vi "PID engine.vi"(0 "Temp In (deg C)":dbl format="%.2f", 7 "Control Parameters":T1={"Setpoint"=50.0, "Control bandwidth"=4.0, "Settle bandwidth"=1.0, "Integral time"=30.0, "Int\non"=TRUE, "Derivative time"=0.5, "Der\non"=FALSE, "Settle time"=200.0} {"Settle time" format="%.2f"; "Derivative time" format="%.2f"; "Integral time" format="%.2f"; "Settle bandwidth" format="%.2f"; "Control bandwidth" format="%.2f"; "Setpoint" format="%.2f"}, 11 "error in":errorcluster, 12 "Normalized Power In (0-1)":dbl format="%.2f", 13 "index (0=init)":i32, 14 "Manual Override":bool) -> (2 "settled":bool, 3 "time in settle band":dbl format="%.2f", 4 "Normalized Power Out (0-1)":dbl format="%.2f", 15 "error out":errorcluster)   [LabVIEW 2016]
doc: "This VI does the PID calculation.\n\nPaul K Dixon\nPhysics 350\nCSUSB Physics"
uses:
  typedefs/control parameters.ctl
  globals/temp control global variables.vi
panel:
  # "PID Engine"
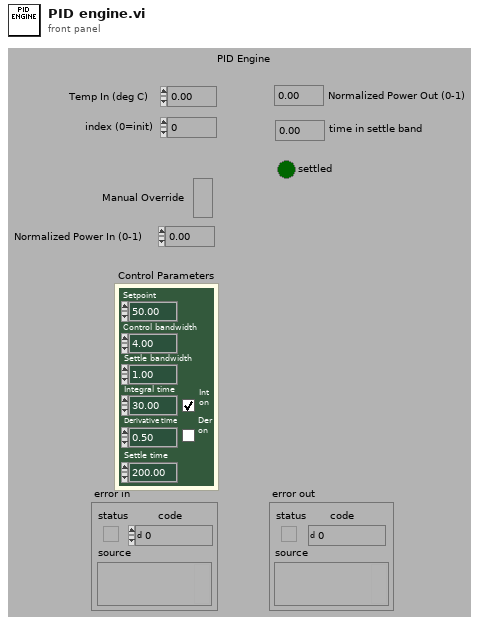
[diagram p1: front panel]
types:
  T1 = typedef "control parameters.ctl" = cluster{"Setpoint":dbl, "Control bandwidth":dbl, "Settle bandwidth":dbl, "Integral time":dbl, "Int\non":bool, "Derivative time":dbl, "Der\non":bool, "Settle time":dbl}
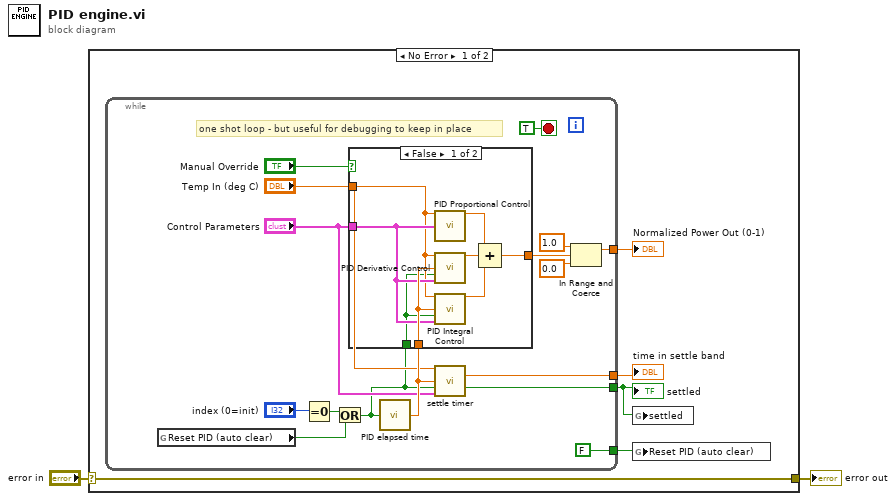
[diagram p0: block diagram]
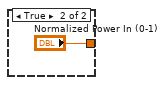
[diagram p2: hidden frame]
diagram:
  n1 = case shown="No Error" "error in" {
    selector: "error in" -> [w5 w33]
    tunnel: [w5 w33] -> w1
    frame No Error {
      n2 = while {
        tunnel: [FALSE ("Reset PID (auto clear)")] -> w4
        tunnel: [w18] -> w3
        tunnel: [w19] -> w6
        tunnel: [w20] -> w7
        stop <- TRUE stop-if-true
        # "one shot loop - but useful for debugging to keep in place"
        n3 = global read "temp control global variables.vi" "Reset PID (auto clear)"() -> (w8:bool)
        n4 = Equal To 0?(x="index (0=init)") -> (x = 0?=w13:bool)
        n5 = Or(x=w13, y=w8) -> (x .or. y?=w10:bool)
        n6 = call "PID elapsed time.vi"("initialize"=w10) -> ("elapsed time"=w15:dbl)  [unwired: 14 out]
        n7 = case shown="False" "Manual Override" {
          tunnel: [w31 "Normalized Power In (0-1)"] -> w21
          tunnel: w15 -> [w27 _]
          tunnel: "Control Parameters" -> [w26 _]
          tunnel: "Temp In (deg C)" -> [w25 _]
          tunnel: w10 -> [w24 _]
          frame False {
            n8 = call "PID Proportional Control.vi"("Temp"=w25, "Control Parameters"=w26) -> ("P Power"=w29:dbl)  [unwired: 1 in, 12 out]
            n9 = call "PID Derivative Control.vi"("Temp In (deg C)"=w25, "time interval"=w27, "initialize"=w24, "Control Parameters"=w26) -> ("Derivative Power"=w30:dbl)  [unwired: 1 in, 10 out]
            n10 = call "PID Integral Control.vi"("Temp In (deg C)"=w25, "time interval"=w27, "initialize"=w24, "Control Parameters"=w26) -> ("Integral Power"=w28:dbl)  [unwired: 1 in, 10 out]
            n11 = Compound Arithmetic op=ADD(w29, w30, w28) -> (w31:dbl)
          }
          frame True {
          }
        }
        n12 = call "settle timer.vi"("Temp In (deg C)"="Temp In (deg C)", "elapsed time"=w15, "initialize"=w10, "Control Parameters"="Control Parameters") -> ("time in settle band"=w19:dbl, "settled"=w18:bool)  [unwired: 3 in, 7 out]
        n13 = In Range and Coerce(upper limit=1.0, x=w21, lower limit=0.0) -> (coerced(x)=w20:dbl)  [unwired: 1 out]
      }
      "settled" <- w3
      "time in settle band" <- w6
      "Normalized Power Out (0-1)" <- w7
      n14 = global write "temp control global variables.vi" "settled"(w3) -> ()
      n15 = global write "temp control global variables.vi" "Reset PID (auto clear)"(w4) -> ()
    }
    frame Error {
    }
  }
  "error out" <- w1
